vi "Lazo_for.vi"() -> ()   [LabVIEW 2020]
panel:
  out "number (0 to 1)":dbl
  out "i":i32
  in  "Control de iteración":i32
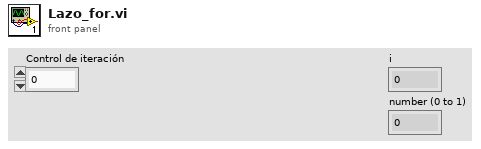
[diagram p1: front panel]
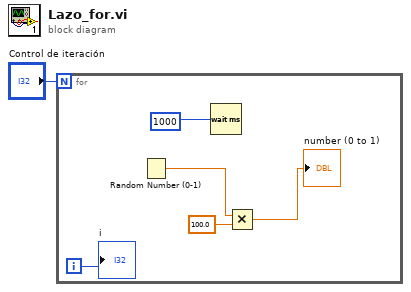
[diagram p0: block diagram]
diagram:
  n1 = for {
    N: "Control de iteración" -> [_]
    i -> [w6]
    n2 = Random Number (0-1)() -> (number: 0 to 1=w4:dbl)
    n3 = Wait (ms)(milliseconds to wait=u32 1000 ("millisecond timer value")) -> ()  [unwired: 1 out]
    n4 = Multiply(x=w4, y=100.0) -> (x*y=→"number (0 to 1)":dbl)
    "i" <- w6
  }
